vi "lv stream sample.vi"() -> ()   [LabVIEW 2026]
uses:
  lv deref string.vi
  <vilib>/Utility/error.llb/Error Cluster From Error Code.vi
  bin/nominalClient_64.dll
panel:
  out "error out":errorcluster
  in  "api token":string
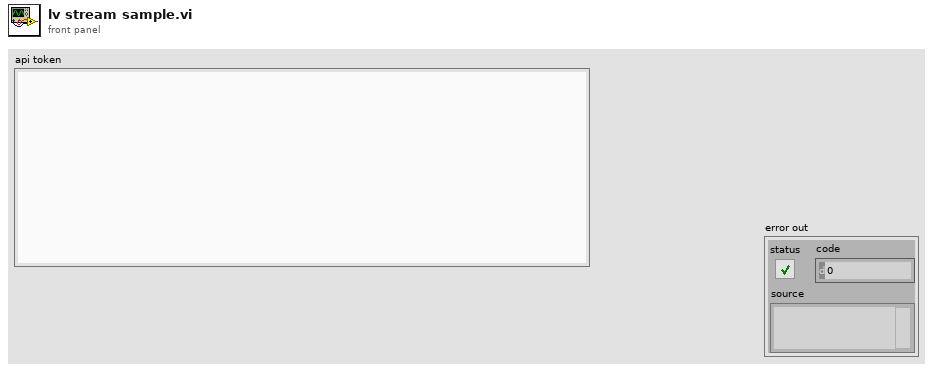
[diagram p1: front panel]
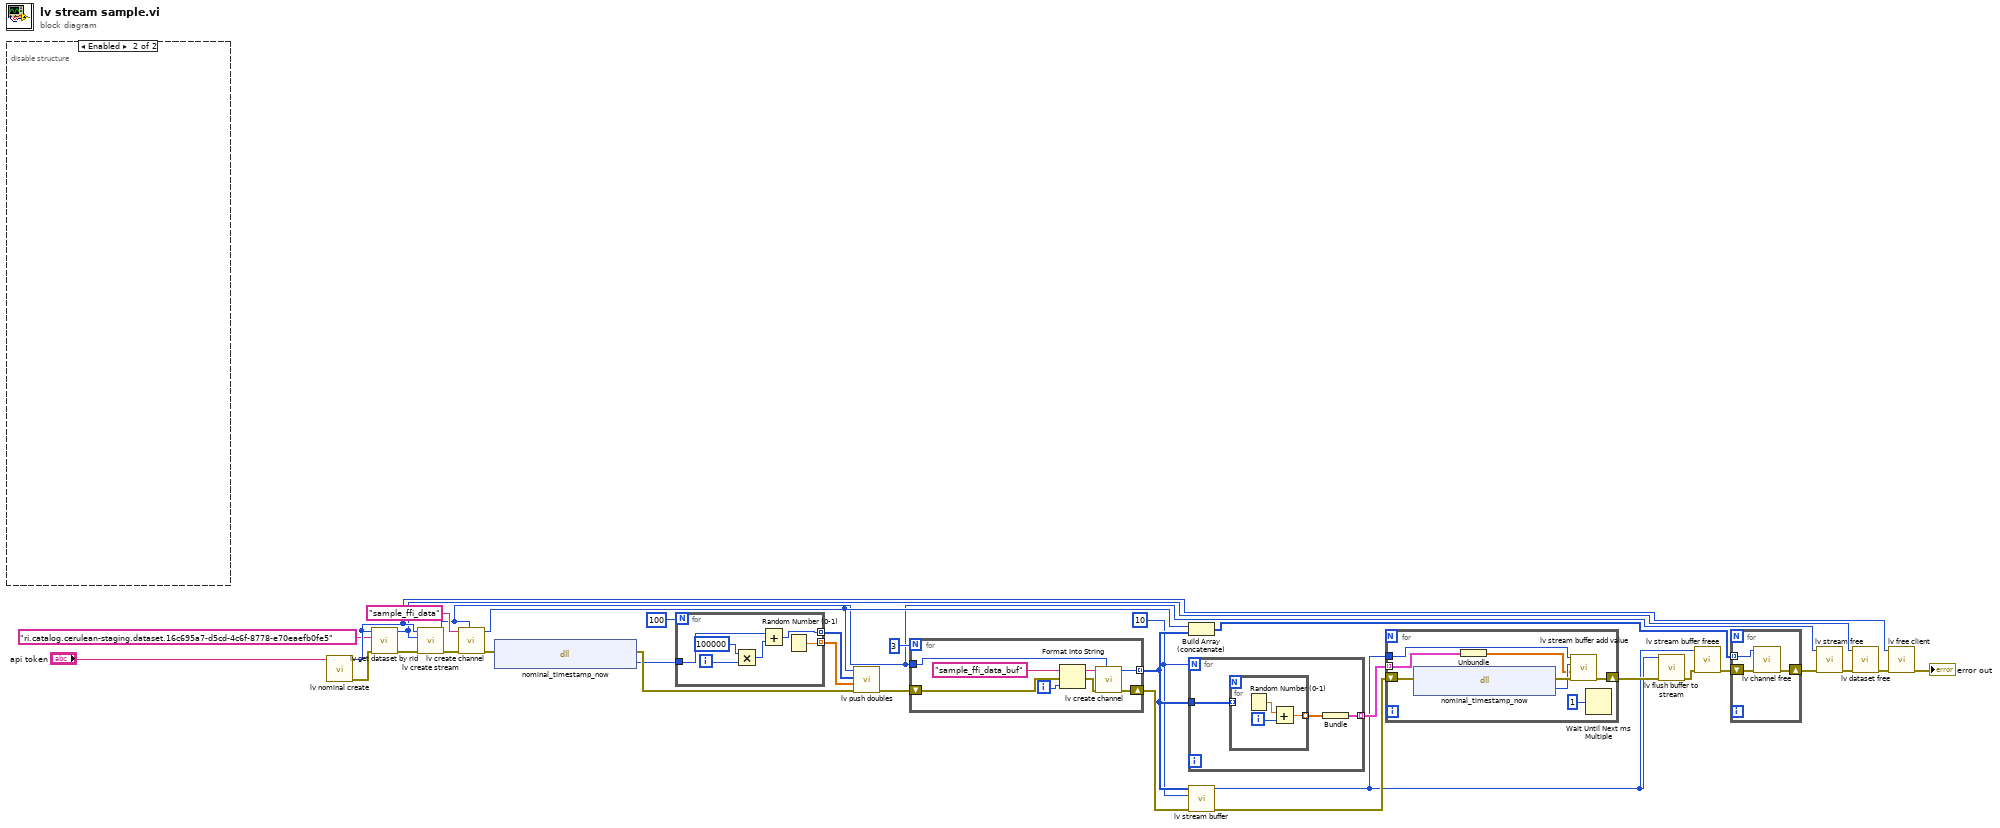
[diagram p0: block diagram]
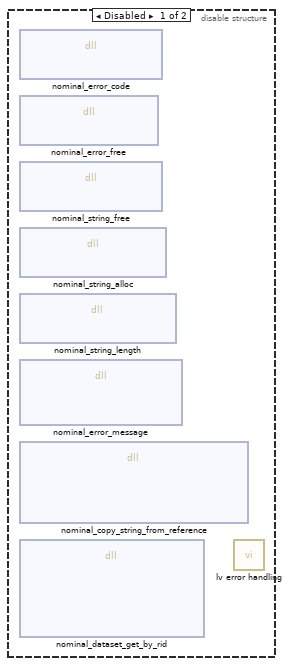
[diagram p2: hidden frame]
diagram:
  w4 = u32 10 ("capacity")
  n1 = disable-structure shown="Enabled" {
    frame Disabled {
      n2 = dll-call lib="C:/sw/nominal-c/bin/nominalClient_64.dll" fn="nominal_error_code"() -> ()  [unwired: 6 in, 2 out]
      n3 = dll-call lib="C:/sw/nominal-c/bin/nominalClient_64.dll" fn="nominal_error_free"() -> ()  [unwired: 6 in, 2 out]
      n4 = dll-call lib="C:/sw/nominal-c/bin/nominalClient_64.dll" fn="nominal_string_free"() -> ()  [unwired: 6 in, 2 out]
      n5 = dll-call lib="C:/sw/nominal-c/bin/nominalClient_64.dll" fn="nominal_string_alloc"() -> ()  [unwired: 6 in, 2 out]
      n6 = dll-call lib="C:/sw/nominal-c/bin/nominalClient_64.dll" fn="nominal_string_length"() -> ()  [unwired: 6 in, 2 out]
      n7 = dll-call lib="C:/sw/nominal-c/bin/nominalClient_64.dll" fn="nominal_error_message"() -> ()  [unwired: 8 in, 2 out]
      n8 = dll-call lib="C:/sw/nominal-c/bin/nominalClient_64.dll" fn="nominal_copy_string_from_reference"() -> ()  [unwired: 10 in, 2 out]
      n9 = dll-call lib="C:/sw/nominal-c/bin/nominalClient_64.dll" fn="nominal_dataset_get_by_rid"() -> ()  [unwired: 12 in, 2 out]
      n10 = call "lv error handling.vi"() -> ()  [unwired: 11 in, 1 out]
    }
    frame Enabled {
    }
  }
  n11 = call "lv nominal create.vi"("api token"="api token") -> ("error out"=w31:errorcluster, "client handle"=w27:i32)  [unwired: 9 in]
  n12 = call "lv get dataset by rid.vi"("error in"=w31, "dataset rid"="ri.catalog.cerulean-staging.dataset.16c695a7-d5cd-4c6f-8778-e70eaefb0fe5" ("workspace rid"), "client handle"=w27) -> ("error out"=w29:errorcluster, "dataset handle"=w10:i32)  [unwired: 7 in]
  n13 = call "lv create stream.vi"("error in"=w29, "dataset handle"=w10, "client handle"=w27) -> ("error out"=w28:errorcluster, "stream handle"=w2:i32)  [unwired: 7 in]
  n14 = call "lv create channel.vi"("stream"=w2, "error in (no error)"=w28, "name"="sample_ffi_data") -> ("error out"=w25:errorcluster, "channel handle"=w15:i32)  [unwired: 7 in]
  n15 = dll-call lib="C:/sw/nominal-c/bin/nominalClient_64.dll" fn="nominal_timestamp_now"(error in=w25) -> (error out=w24:errorcluster, "timestamp"=w22:i64)  [unwired: 2 in, 1 out]
  n16 = for {
    N: 100 -> [_]
    tunnel: [w38] -> w20 mode=indexing
    tunnel: w22 -> [w35]
    tunnel: [w33] -> w21 mode=indexing
    i -> [w37]
    n17 = Multiply(x=100000, y=w37) -> (x*y=w36:i32)
    n18 = Add(x=w35, y=w36) -> (x+y=w33:i64)
    n19 = Random Number (0-1)() -> (number: 0 to 1=w38:dbl)
  }
  n20 = call "lv push doubles.vi"("error in"=w24, "values"=w20, "timestamps (ns)"=w21, "channel handle"=w15) -> ("error out"=w19:errorcluster)  [unwired: 7 in]
  n21 = for {
    N: 3 -> [_]
    shift-right: [w45] -> w18
    shift-left: w19 -> [w46]
    tunnel: [w40] -> w5 mode=indexing
    tunnel: w2 -> [w39]
    i -> [w42]
    n22 = Format Into String(initial string="sample_ffi_data_buf" ("name"), error in=w46, w42) -> (resulting string=w41:string, error out=w44:errorcluster)  [unwired: 1 in]
    n23 = call "lv create channel.vi"("stream"=w39, "error in (no error)"=w44, "name"=w41) -> ("error out"=w45:errorcluster, "channel handle"=w40:i32)  [unwired: 7 in]
  }
  n24 = Build Array (concatenate)(w15, w5) -> (w14:i32[])
  n25 = for {
    N: w4 -> [_]
    tunnel: w5 -> [w49]
    tunnel: [w47] -> w3 mode=indexing
    n26 = for {
      tunnel: [w50] -> w48 mode=indexing
      tunnel: w49 -> [_] mode=indexing
      i -> [w51]
      n27 = Random Number (0-1)() -> (number: 0 to 1=w52:dbl)
      n28 = Add(x=w52, y=w51) -> (x+y=w50:dbl)
    }
    n29 = Bundle(w48) -> (w47:cluster{dbl[]})  [unwired: 1 in]
  }
  n30 = call "lv stream buffer.vi"("error in"=w18, "size per ch"=w4, "channels"=w5) -> ("error out"=w9:errorcluster, "buffer handle"=w1:i32)  [unwired: 7 in]
  n31 = for {
    shift-right: [w60] -> w8
    shift-left: w9 -> [w58]
    tunnel: w1 -> [w59]
    tunnel: w3 -> [w55] mode=indexing
    n32 = dll-call lib="C:/sw/nominal-c/bin/nominalClient_64.dll" fn="nominal_timestamp_now"(error in=w58) -> (error out=w57:errorcluster, "timestamp"=w56:i64)  [unwired: 2 in, 1 out]
    n33 = Unbundle(w55) -> (w54:dbl[])
    n34 = call "lv stream buffer add value.vi"("error in"=w57, "data values"=w54, "timestamp"=w56, "buffer handle"=w59) -> ("error out"=w60:errorcluster)  [unwired: 6 in, 1 out]
    n35 = Wait Until Next ms Multiple(millisecond multiple=u32 1) -> ()  [unwired: 1 out]
  }
  n36 = call "lv flush buffer to stream.vi"("error in"=w8, "buffer handle"=w1) -> ("error out"=w7:errorcluster)  [unwired: 9 in]
  n37 = call "lv stream buffer freee.vi"("error in"=w7, "buffer handle"=w1) -> ("error out"=w16:errorcluster)  [unwired: 9 in]
  n38 = for {
    shift-right: [w62] -> w12
    shift-left: w16 -> [w63]
    tunnel: w14 -> [w61] mode=indexing
    n39 = call "lv channel free.vi"("error in (no error)"=w63, "channel handle"=w61) -> ("error out"=w62:errorcluster)  [unwired: 9 in]
  }
  n40 = call "lv stream free.vi"("error in"=w12, "stream handle"=w2) -> ("error out"=w11:errorcluster)  [unwired: 9 in]
  n41 = call "lv dataset free.vi"("error in"=w11, "dataset handle"=w10) -> ("error out"=w13:errorcluster)  [unwired: 9 in]
  n42 = call "lv free client.vi"("error in"=w13, "client handle"=w27) -> ("error out"=→"error out":errorcluster)  [unwired: 9 in]
